vi "FindSymbol.vi"(8 "error in (no error)":errorcluster, 10 "pattern":string="开发环境 *", 11 "path":path=path "D:/projects/Multi-LabVIEW-Selector/support") -> (0 "error out":errorcluster, 1 "Version":string, 2 "Exits?":bool, 3 "path (dup)":path, 4 "found path":path)   [LabVIEW 2014]
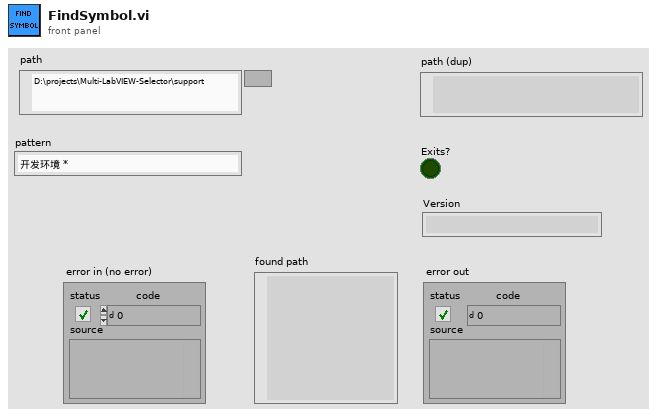
[diagram p1: front panel]
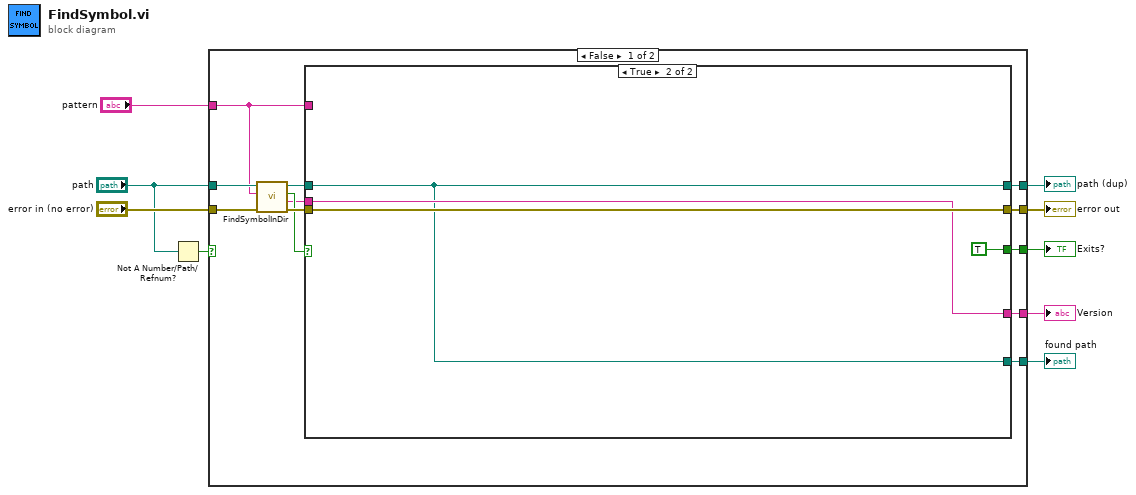
[diagram p0: block diagram]
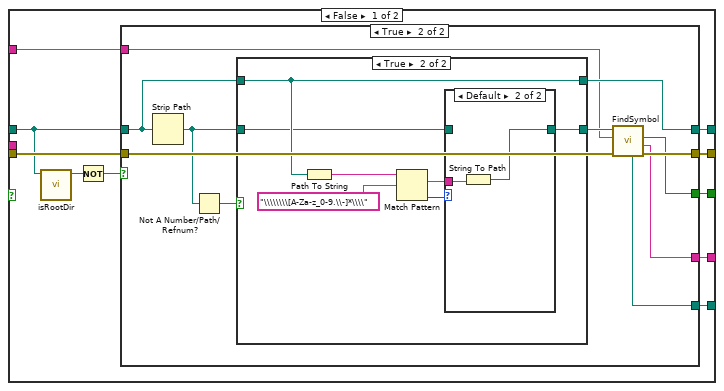
[diagram p2: hidden frame]
diagram:
  n1 = Not A Number/Path/Refnum?(number/path/refnum="path") -> (NaN/Path/Refnum?=w2:bool)
  n2 = case shown="False" w2 {
    tunnel: "error in (no error)" -> [w21 w61]
    tunnel: [w18 w62] -> w8
    tunnel: [w17 _] -> w7
    tunnel: [w16 w61] -> w6
    tunnel: [w15 _] -> w5
    tunnel: [w12 _] -> w4
    tunnel: "path" -> [w11 w62]
    tunnel: "pattern" -> [w10 _]
    frame False {
      n3 = call "FindSymbolInDir.vi"("error in (no error)"=w21, "pattern"=w10, "path"=w11) -> ("error out"=w19:errorcluster, "String"=w13:string, "Exits?"=w14:bool, "path (dup)"=w20:path)  [unwired: 5 in]
      n4 = case shown="True" w14 {
        tunnel: w20 -> [w26 w57]
        tunnel: w19 -> [w31 w60]
        tunnel: [w30 w57] -> w18
        tunnel: [w29 TRUE ("Exits?")] -> w17
        tunnel: [w28 w60] -> w16
        tunnel: [w27 w59] -> w15
        tunnel: w13 -> [_ w59]
        tunnel: [w23 w57] -> w12
        tunnel: w10 -> [w22 _]
        frame False {
          n5 = call "isRootDir.vi"("path"=w26) -> ("Boolean"=w25:bool)  [unwired: 10 in]
          n6 = Not(x=w25) -> (.not. x?=w24:bool)
          n7 = case shown="True" w24 {
            tunnel: w26 -> [w33 w36]
            tunnel: w31 -> [w32 w44]
            tunnel: [w32 w43] -> w28
            tunnel: [w33 w35] -> w30
            tunnel: [_ w42] -> w29
            tunnel: [_ w41] -> w27
            tunnel: [_ w40] -> w23
            tunnel: w22 -> [_ w34]
            frame False {
            }
            frame True {
              n8 = Strip Path(path=w36) -> (stripped path=w37:path)  [unwired: 1 out]
              n9 = Not A Number/Path/Refnum?(number/path/refnum=w37) -> (NaN/Path/Refnum?=w39:bool)
              n10 = case shown="True" w39 {
                tunnel: w37 -> [w46 w47]
                tunnel: [w46 w50] -> w38
                tunnel: w36 -> [w45 w48]
                tunnel: [w45 w48] -> w35
                frame False {
                }
                frame True {
                  n11 = Path To String(path=w48) -> (string=w52:string)
                  n12 = Match Pattern(string=w52, regular expression="\\\\\\\\[A-Za-z_0-9.\\-]*\\\\") -> (match substring=w51:string, offset past match=w49:i32)  [unwired: 1 in, 2 out]
                  n13 = case shown="Default" w49 {
                    tunnel: w51 -> [_ w56]
                    tunnel: [w54 w55] -> w50
                    tunnel: w47 -> [w54 _]
                    frame -1 {
                    }
                    frame Default {
                      n14 = String To Path(string=w56) -> (path=w55:path)
                    }
                  }
                }
              }
              n15 = call "FindSymbol.vi"("error in (no error)"=w44, "pattern"=w34, "path"=w38) -> ("error out"=w43:errorcluster, "Version"=w41:string, "Exits?"=w42:bool, "found path"=w40:path)  [unwired: 4 in, 1 out]
            }
          }
        }
        frame True {
        }
      }
    }
    frame True {
    }
  }
  "error out" <- w6
  "Exits?" <- w7
  "Version" <- w5
  "path (dup)" <- w8
  "found path" <- w4
